vi "Newport ITX-D3N IBTHX Data.vi"(7 "Disable Filter?":bool=TRUE, 8 "error in (no error)":errorcluster, 11 "TCP Network Connection in":refnum<k5>) -> (0 "error out":errorcluster, 2 "iBTHX Data":T1, 3 "TCP Network Connection out":refnum<k5>)   [LabVIEW 2023]
uses:
  Type Definitions/iBTHX Data Values.ctl
  Type Definitions/iBTHX.ctl
panel:
  out "appended array":bool[](array[boolean])
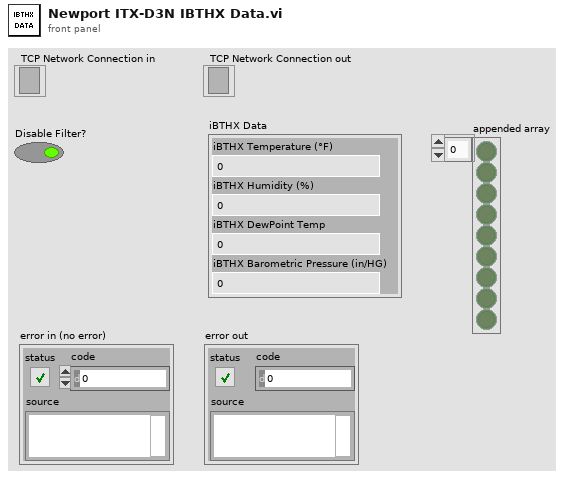
[diagram p1: front panel]
types:
  T1 = typedef "iBTHX Data Values.ctl" = cluster{"iBTHX Barometric Pressure (in/HG)":dbl, "iBTHX Humidity (%)":dbl, "iBTHX Temperature (°F)":dbl, "iBTHX DewPoint Temp":dbl}
  T2 = typedef "iBTHX.ctl" = string
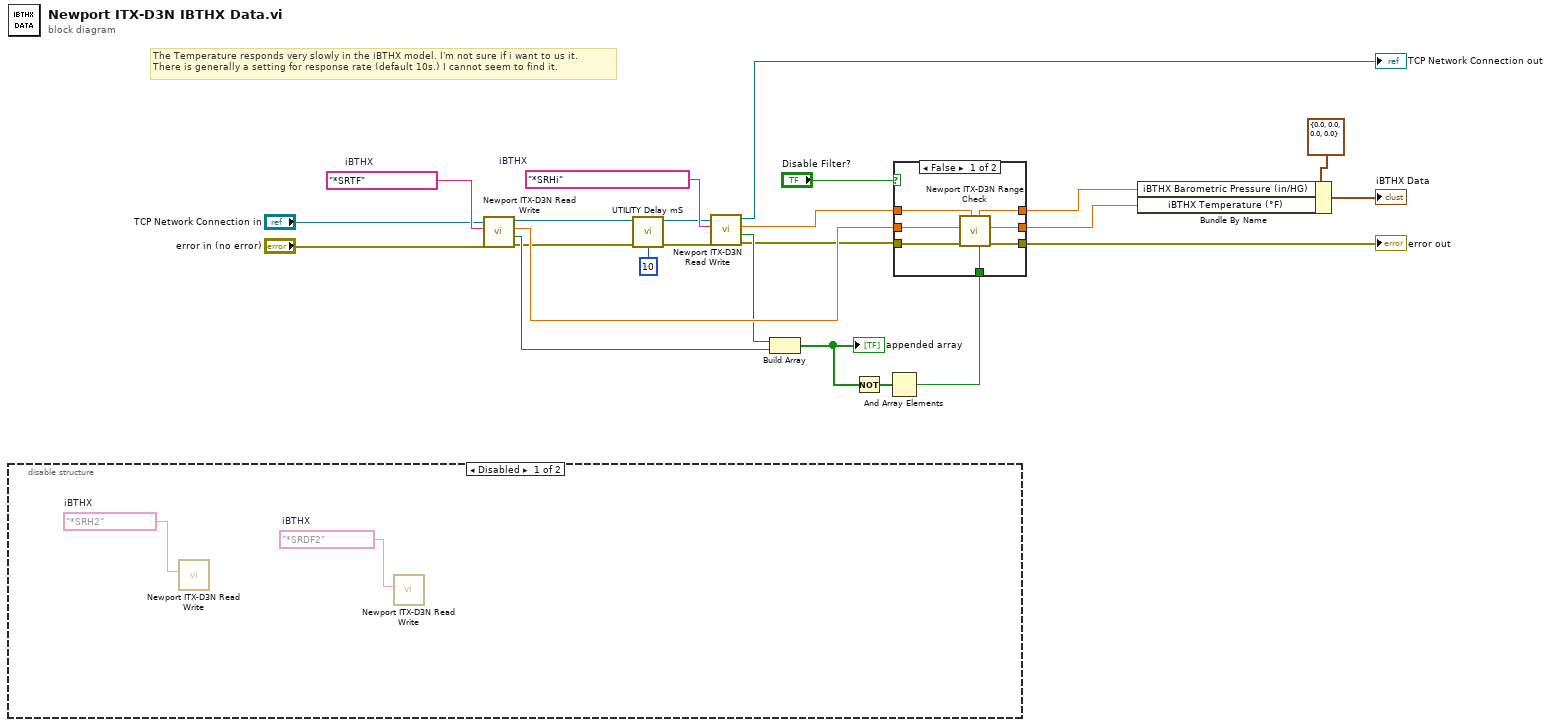
[diagram p0: block diagram]
diagram:
  w23 = T2 "*SRTF"  # iBTHX
  w22 = T2 "*SRHi"  # iBTHX
  # "The Temperature responds very slowly in the iBTHX model. I'm not sure if i want to us it.\nThere is generally a setting for response rate (default 10s.) I cannot seem to find it."
  n1 = disable-structure shown="Disabled" {
    frame Disabled {
      w24 = T2 "*SRDF2"  # iBTHX
      w25 = T2 "*SRH2"  # iBTHX
      n2 = call "Newport ITX-D3N Read Write.vi"("iTHX Commands"=w25) -> ()  [unwired: 7 in, 4 out]
      n3 = call "Newport ITX-D3N Read Write.vi"("iTHX Commands"=w24) -> ()  [unwired: 7 in, 4 out]
    }
    frame Enabled {
    }
  }
  n4 = call "Newport ITX-D3N Read Write.vi"("error in (no error)"="error in (no error)", "iTHX Commands"=w23, "TCP Network Connection in"="TCP Network Connection in") -> ("error out"=w10:errorcluster, "In Range?"=w13:bool, "Output Data"=w18:dbl, "TCP Network Connection out"=w4:refnum<k5>)  [unwired: 5 in]
  n5 = call "UTILITY Delay mS.vi"("Error In"=w10, "milliseconds to wait"=u32 10) -> ("Error Out"=w2:errorcluster)  [unwired: 13 in]
  n6 = call "Newport ITX-D3N Read Write.vi"("error in (no error)"=w2, "iTHX Commands"=w22, "TCP Network Connection in"=w4) -> ("error out"=w12:errorcluster, "In Range?"=w14:bool, "Output Data"=w16:dbl, "TCP Network Connection out"=→"TCP Network Connection out":refnum<k5>)  [unwired: 5 in]
  n7 = Build Array(w14, w13) -> (w7:bool[])
  "appended array" <- w7
  n8 = Not(x=w7) -> (.not. x?=w8:bool[])
  n9 = And Array Elements(Boolean array=w8) -> (logical AND=w6:bool)
  n10 = case shown="False" "Disable Filter?" {
    tunnel: w18 -> [w32 w34]
    tunnel: [w31 w34] -> w17
    tunnel: w16 -> [w30 w35]
    tunnel: [w29 w35] -> w15
    tunnel: w12 -> [w28 w33]
    tunnel: [w27 w33] -> w11
    tunnel: w6 -> [w26 _]
    frame False {
      n11 = call "Newport ITX-D3N Range Check.vi"("All Out of Range?"=w26, "Barometric Pressure"=w30, "Error In"=w28, "Temperature"=w32) -> ("Error Out"=w27:errorcluster, "Temperature Out"=w31:dbl, "Barometric Pressure Out"=w29:dbl)  [unwired: 3 in, 2 out]
    }
    frame True {
    }
  }
  "error out" <- w11
  n12 = Bundle By Name(cluster=T1 {"iBTHX Barometric Pressure (in/HG)"=0.0, "iBTHX Humidity (%)"=0.0, "iBTHX Temperature (°F)"=0.0, "iBTHX DewPoint Temp"=0.0} ("iBTHX"), "iBTHX Barometric Pressure (in/HG)"=w15, "iBTHX Temperature (°F)"=w17) -> (→"iBTHX Data":T1)
